vi "Create Report Path.vi"(8 "error in (no error)":errorcluster, 11 "Report Generator in":refnum<class "Report Generator.lvclass">) -> (0 "error out":errorcluster, 2 "Unique Test Name":string, 3 "Report Generator out":refnum<class "Report Generator.lvclass">)   [LabVIEW 2023, in "Report Generator.lvlib" / "Report Generator.lvclass"]
doc: "Create Test Directory:\n\n<Default Data Directory>\\Model\\Serial\\Testname\n\nThis ensures that all test data is organized by the unit under test, and the tests performed on the unit.\n\nThe <b>Unique Test Name</b> in path creation is the testname with a date time component appended so duplicate tests can be performed on the same unit."
uses:
  Library/Report Generator.lvclass
  C:/Users/Public/Documents/Development/builds/Framework/Engine.lvlibp/Engine/Library/Engine.lvclass
  builds/Framework/Engine.lvlibp/Engine/Accessors/DVRs/Read Model.vi
  builds/Framework/Engine.lvlibp/Engine/Accessors/DVRs/Read Serial.vi
  builds/Framework/Engine.lvlibp/Engine/Accessors/DVRs/Read TestName.vi
  builds/Framework/Engine.lvlibp/Engine/Accessors/DVRs/Write ReportDir.vi
  Library/Report Generator.lvclass/Report Generator.ctl
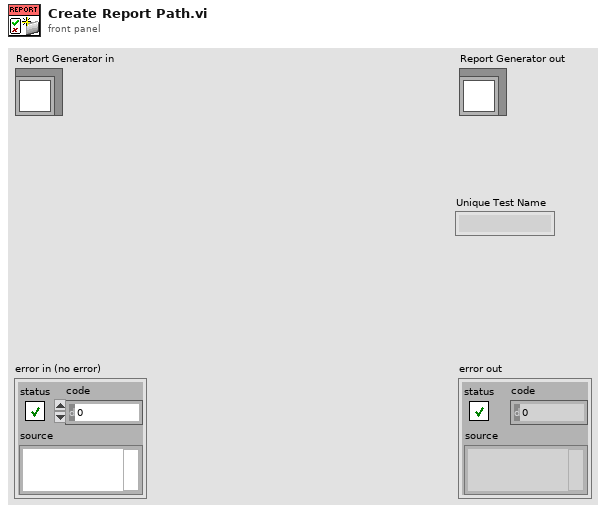
[diagram p1: front panel]
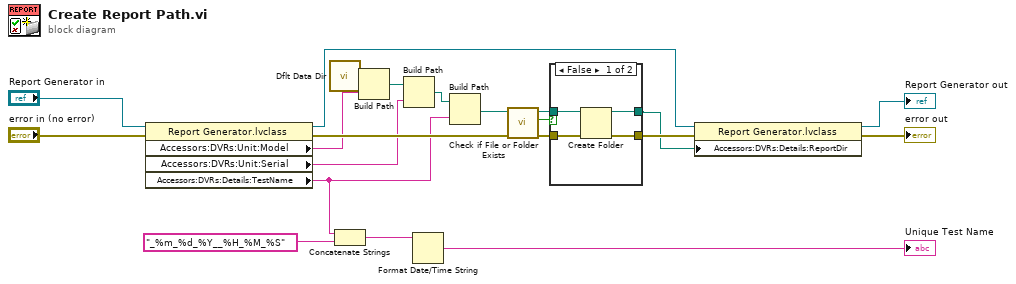
[diagram p0: block diagram]
diagram:
  n1 = property class="Report Generator.lvclass"(reference="Report Generator in", error in="error in (no error)") -> (reference out=w9:refnum<class "Report Generator.lvclass">, error out=w15:errorcluster, "Accessors:DVRs:Unit:Model"=w12:string, "Accessors:DVRs:Unit:Serial"=w11:string, "Accessors:DVRs:Details:TestName"=w1:string)
  n2 = call <vilib>:"Dflt Data Dir.vi"() -> ("App:Default Data Directory"=w16:path)
  n3 = Concatenate Strings(w1, "_%m_%d_%Y__%H_%M_%S" ("time format string (%c)")) -> (w3:string)
  n4 = Build Path(base path=w16, name or relative path=w12) -> (appended path=w19:path)
  n5 = Build Path(base path=w19, name or relative path=w11) -> (appended path=w6:path)
  n6 = Format Date/Time String(time format string (%c)=w3) -> (date/time string=→"Unique Test Name":string)  [unwired: 2 in]
  n7 = Build Path(base path=w6, name or relative path=w1) -> (appended path=w5:path)
  n8 = call <vilib>:"Check if File or Folder Exists.vi"("error in (no error)"=w15, "path"=w5) -> ("error out"=w14:errorcluster, "file or folder exists?"=w18:bool, "dup path"=w17:path)  [unwired: 7 in]
  n9 = case shown="False" w18 {
    tunnel: w17 -> [w25 w27]
    tunnel: [w24 w27] -> w7
    tunnel: w14 -> [w23 w26]
    tunnel: [w22 w26] -> w13
    frame False {
      n10 = Create Folder(path (use dialog)=w25, error in=w23) -> (created path=w24:path, error out=w22:errorcluster)  [unwired: 1 in, 1 out]
    }
    frame True {
    }
  }
  n11 = property class="Report Generator.lvclass"(reference=w9, error in=w13, "Accessors:DVRs:Details:ReportDir"=w7) -> (reference out=→"Report Generator out":refnum<class "Report Generator.lvclass">, error out=→"error out":errorcluster)
